vi "car_state_driver.vi"(1 "START":dbl, 2 "RTDS":dbl, 3 "ON":dbl, 4 "OFF":dbl) -> (0 "Car State":string)   [LabVIEW 2017]
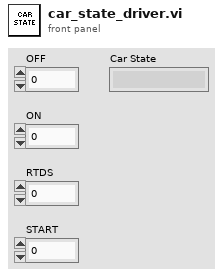
[diagram p1: front panel]
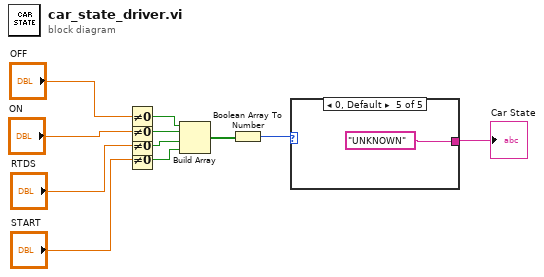
[diagram p0: block diagram]
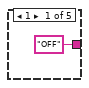
[diagram p2: hidden frame]
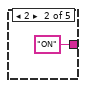
[diagram p3: hidden frame]
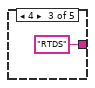
[diagram p4: hidden frame]
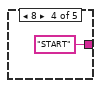
[diagram p5: hidden frame]
diagram:
  n1 = Not Equal To 0?(x="OFF") -> (x != 0?=w4:bool)
  n2 = Not Equal To 0?(x="ON") -> (x != 0?=w5:bool)
  n3 = Not Equal To 0?(x="RTDS") -> (x != 0?=w6:bool)
  n4 = Not Equal To 0?(x="START") -> (x != 0?=w7:bool)
  n5 = Build Array(w4, w5, w6, w7) -> (w1:bool[])
  n6 = Boolean Array To Number(Boolean array=w1) -> (number=w2:u32)
  n7 = case shown="0, Default" w2 {
    tunnel: ["OFF" "ON" "RTDS" "START" "UNKNOWN"] -> w3
    frame 1 {
    }
    frame 2 {
    }
    frame 4 {
    }
    frame 8 {
    }
    frame 0, Default {
    }
  }
  "Car State" <- w3
